vi "Set TWM Measurement.vi"(7 "Measurement properties":T1={"Measurement ID"=enum."1", "Description"="3 phase, 3 ADC, 1 PJVS", "Switching matrix M"=[], "Signal frequency  (Hz)"=50.0, "Signal amplitudes (V)"=[1.0, 1.0], "PRs (s)"=0.0, "PRe (s)"=0.0, "MRs (s)"=0.0, "MRe (s)"=0.0, "Set PJVS frequency (Hz)"=50.0, "PJVS reference voltages (1 period, V)"=[], "Requiested PJVS steps"=10, "Sampling f (Hz)"=7000.0, "Trigger mode"=enum."Trigger every MX switch", "Timing matrix (periods)"=[], "Record length (multiples of M)"=1, "Calculated"={"Triggers to next path (line of sequence)"=[], "Record samples"=0, "Sample indexes of switches"=[], "PRs (samples)"=0, "PRe (samples)"=0, "MRs (samples)"=0, "MRe (samples)"=0, "Trigger frequency  (Hz)"=50.0, "Measurement druation (s)"=0.0}} {"Calculated"."Trigger frequency  (Hz)" format="%#_6p"; "Record length (multiples of M)" min=1 step=1; "PJVS reference voltages (1 period, V)" format="%.9g"; "MRe (s)" format="%#_4p"; "MRs (s)" format="%#_4p"; "PRe (s)" format="%#.4p"; "PRs (s)" format="%#_4p"}, 8 "error in":errorcluster, 11 "handle":i32) -> (0 "error out":errorcluster, 3 "handle out":i32)   [LabVIEW 2020]
uses:
  Type definitions/Measuement properties.ctl
  Type definitions/Measurement ID.ctl
  Type definitions/Trigger mode.ctl
  TWM - github/lvprog/octave/infolib/I64.vi
  TWM - github/lvprog/octave/infolib/EXT.vi
  TWM - github/lvprog/octave/infolib/U64.vi
  TWM - github/lvprog/server/TWM client/TWM Client.lvlib
  TWM - github/lvprog/octave/infolib/infolib.lvlib
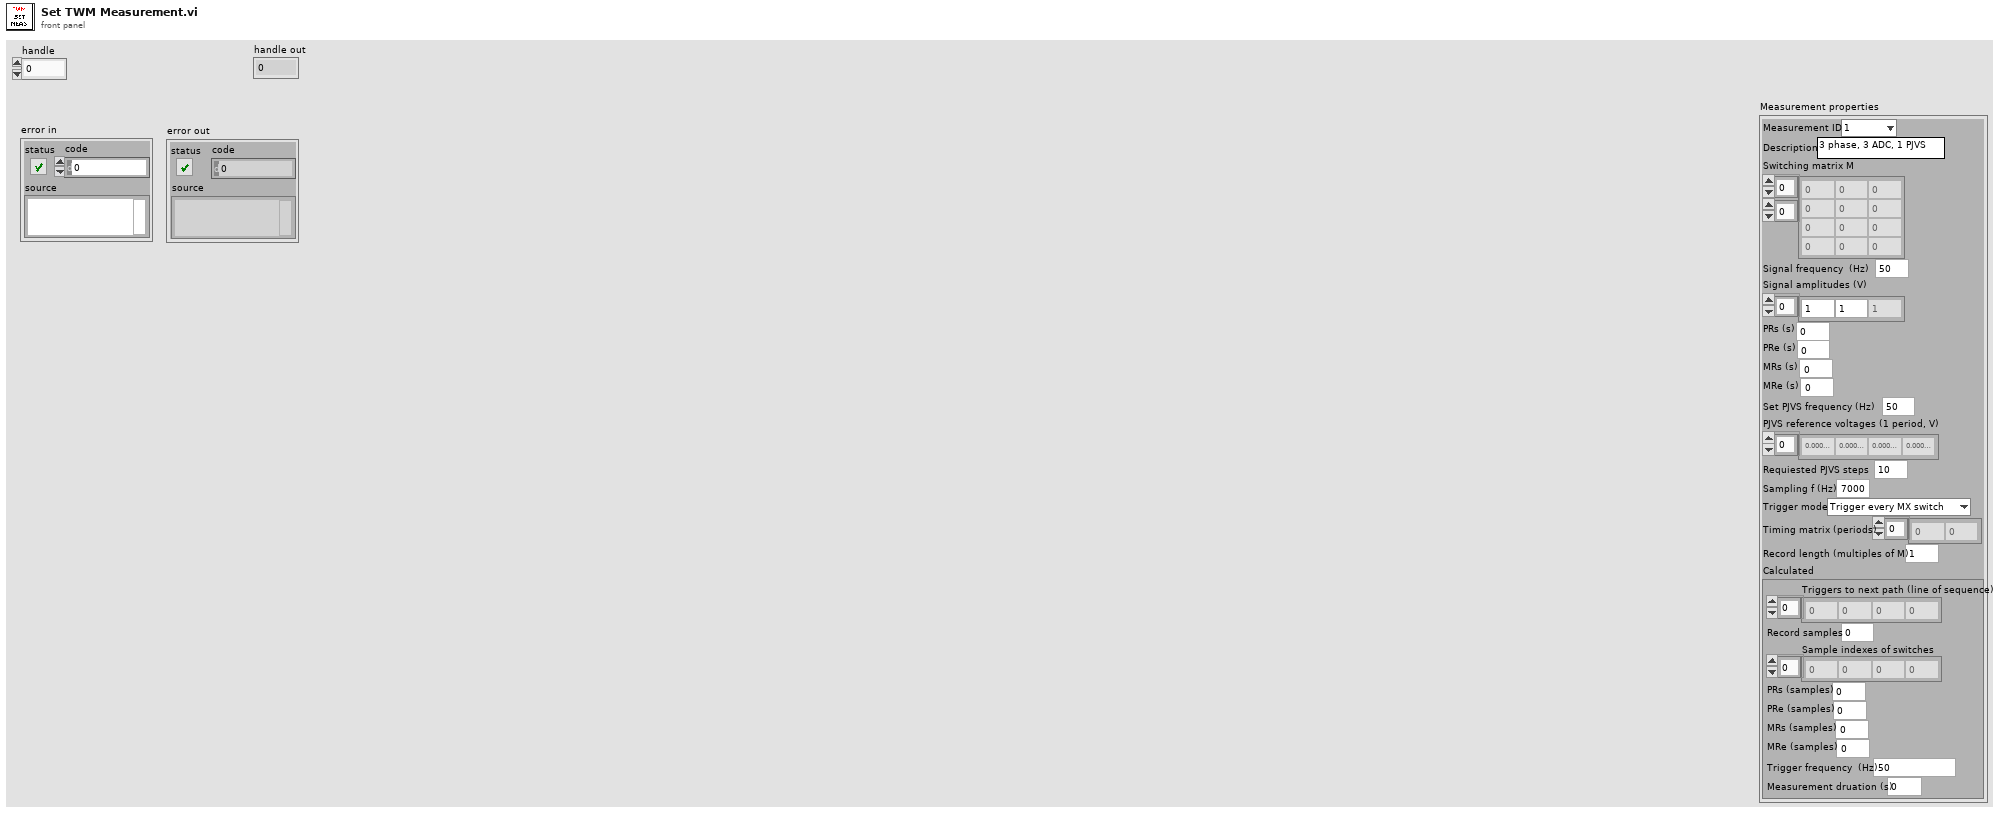
[diagram p1: front panel]
types:
  T1 = typedef "Measuement properties.ctl" = cluster{"Measurement ID":T2, "Description":string, "Switching matrix M":u32[][], "Signal frequency  (Hz)":dbl, "Signal amplitudes (V)":dbl[], "PRs (s)":dbl, "PRe (s)":dbl, "MRs (s)":dbl, "MRe (s)":dbl, "Set PJVS frequency (Hz)":dbl, "PJVS reference voltages (1 period, V)":dbl[], "Requiested PJVS steps":u32, "Sampling f (Hz)":dbl, "Trigger mode":T3, "Timing matrix (periods)":i32[], "Record length (multiples of M)":u32, "Calculated":cluster{"Triggers to next path (line of sequence)":u32[], "Record samples":u32, "Sample indexes of switches":u32[], "PRs (samples)":i32, "PRe (samples)":i32, "MRs (samples)":i32, "MRe (samples)":i32, "Trigger frequency  (Hz)":dbl, "Measurement druation (s)":dbl}}
  T2 = typedef "Measurement ID.ctl" = enum16{"M", "1", "2", "3"}
  T3 = typedef "Trigger mode.ctl" = enum16{"Trigger every MX switch", "Trigger every sample"}
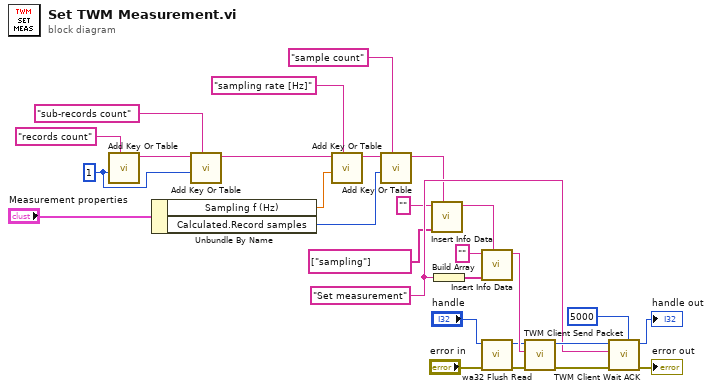
[diagram p0: block diagram]
diagram:
  w7 = 1 ("sub-records")
  w20 = "Set measurement" ("section name")
  n1 = call-poly "Add Key Or Table.vi"("key description"="records count", "numeric"=w7) -> ("info data out"=w12:string)  [unwired: 8 in, 1 out]
  n2 = Unbundle By Name("Measurement properties") -> ("Sampling f (Hz)"=w5:dbl, "Calculated.Record samples"=w2:u32)
  n3 = call-poly "Add Key Or Table.vi"("key description"="sub-records count", "numeric"=w7, "info data"=w12) -> ("info data out"=w4:string)  [unwired: 7 in, 1 out]
  n4 = call-poly "Add Key Or Table.vi"("key description"="sampling rate [Hz]", "numeric"=w5, "info data"=w4) -> ("info data out"=w3:string)  [unwired: 7 in, 1 out]
  n5 = call-poly "Add Key Or Table.vi"("key description"="sample count", "numeric"=w2, "info data"=w3) -> ("info data out"=w1:string)  [unwired: 7 in, 1 out]
  n6 = call "Insert Info Data.vi"("info data to insert"=w1, "sections"=string[] ["sampling"], "info data"="") -> ("info data out"=w11:string)  [unwired: 7 in, 1 out]
  n7 = Build Array(w20) -> (w27:string[])
  n8 = call "Insert Info Data.vi"("info data to insert"=w11, "sections"=w27, "info data"="") -> ("info data out"=w28:string)  [unwired: 7 in, 1 out]
  n9 = call "wa32 Flush Read.vi"("error in"="error in", "handle"="handle") -> ("error out"=w18:errorcluster, "handle out"=w17:i32)  [unwired: 7 in, 1 out]
  n10 = call "TWM Client Send Packet.vi"("error in"=w18, "command string"=w28, "handle"=w17) -> ("error out"=w25:errorcluster, "handle out"=w24:i32)  [unwired: 7 in]
  n11 = call "TWM Client Wait ACK.vi"("timeout [ms] (3000)"=5000 ("timeout [ms] (1000)"), "error in"=w25, "command header"=w20, "handle"=w24) -> ("error out"=→"error out":errorcluster, "handle out"=→"handle out":i32)  [unwired: 6 in]
